vi "Get X and Y.vi"   [LabVIEW 2016, in "xy_utilities.lvlib"]
doc: "Returns the X and Y arrays.\n\nWire data to the data input to determine the polymorphic instance to use or manually select the instance."
uses:
  xy_utilities.lvlib
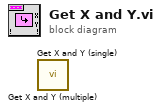
[diagram p0: block diagram]
diagram:
  n1 = call "Get X and Y (multiple).vi"() -> ()  [unwired: 8 in, 4 out]
  n2 = call "Get X and Y (single).vi"() -> ()  [unwired: 8 in, 4 out]
